vi "Test ThermotronDriver.vi"() -> (3 "gRPC Listening Port":i32)   [LabVIEW 2023]
uses:
  Plugin/ThermotronDriver/ThermotronDriver.lvclass
  <vilib>/ADAS Replay HIL/Template Node/Plugin/Template Node/Template Node.lvclass
  <vilib>/ADAS Replay HIL/ADAS Plugin Utilities/AdasLvTemplateSystemLog/AdasLvTemplateSystemLog.lvlib
  <vilib>/ADAS Replay HIL/Template Node/Plugin/Template Node/Common Configuration Params.ctl
  Plugin/ThermotronDriver/Configuration Params.ctl
panel:
  in  "Version":string="1.0"
  in  "Default Parameters":T1={"Common"={"Iteration Interval (s)"=0.001, "T0 (ns)"=0, "Priority"=100, "Processor"=-2, "Wait in Ready State"=TRUE}} {"Common"."Iteration Interval (s)" format="%#_13g"}
  out "# of errors":i32
  in  "stop":bool
  out "Errors":errorcluster[](array[cluster])
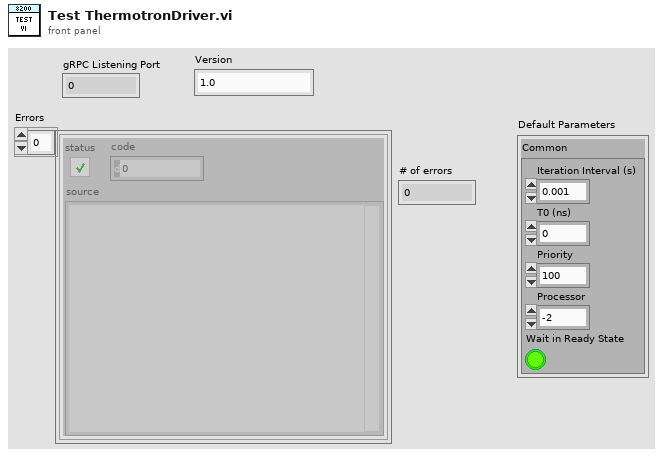
[diagram p1: front panel]
types:
  T1 = typedef "ThermotronDriver.lvlib/ThermotronDriver.lvclass/Configuration Params.ctl" = cluster{"Common":T2}
  T2 = typedef "Template Node.lvlib/Template Node.lvclass/Common Configuration Params.ctl" = cluster{"Iteration Interval (s)":dbl, "T0 (ns)":u64, "Priority":i32, "Processor":i32, "Wait in Ready State":bool}
  T3 = cluster{"Initial Setup":bool, "User Execute":bool, "Sequence Changed":bool, "Continuous Execution":bool, "Block Is Active":bool, "Animating Execution":bool}
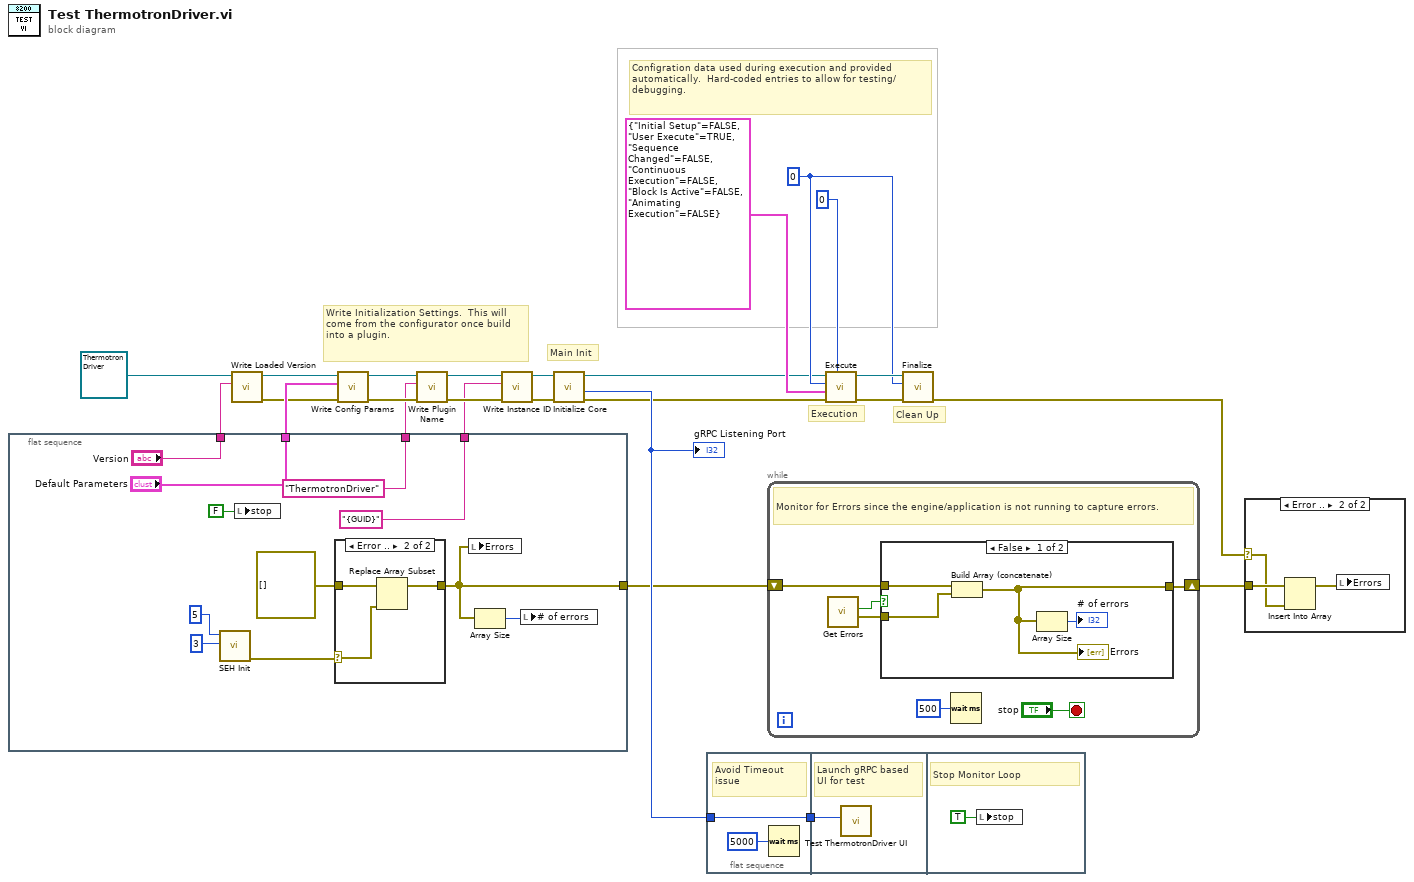
[diagram p0: block diagram]
diagram:
  w14 = u64 0 ("Handle")
  # "Clean Up"
  # "Execution"
  # "Configration data used during execution and provided automatically.  Hard-coded entries to allow for testing/debugging."
  # "Main Init"
  # "Write Initialization Settings.  This will come from the configurator once build into a plugin."
  n1 = flat-sequence {
    tunnel: ["ThermotronDriver" ("Plugin Name")] -> w17
    tunnel: ["{GUID}" ("Instance ID")] -> w16
    tunnel: ["Default Parameters"] -> w11
    tunnel: [w28] -> w8
    tunnel: ["Version"] -> w1
    frame #0 {
      n2 = call <userlib>:"SEH Init.vi"("Number of Priorities"=3, "Notifications per Priority"=5) -> ("error out"=w29:errorcluster)  [unwired: 9 in]
      n3 = local write "stop"(FALSE ("stop")) -> ()
      n4 = case shown="Error .." w29 {
        selector: w29 -> [_ w39]
        tunnel: errorcluster[] [] -> [w37 w40]
        tunnel: [w37 w38] -> w28
        frame No Error {
        }
        frame Error {
          n5 = Replace Array Subset(array=w40, new element=w39) -> (w38:errorcluster[])  [unwired: 1 in]
        }
      }
      n6 = local write "Errors"(w28) -> ()
      n7 = Array Size(array=w28) -> (size(s)=w27:i32)
      n8 = local write "# of errors"(w27) -> ()
    }
  }
  n9 = call <vilib>:"Write Loaded Version.vi"("Loaded Version"=w1, "Template Node in"=refnum<class "ThermotronDriver.lvclass"> refnum ("Test Node.lvlib:Test Node.lvclass")) -> ("error out"=w2:errorcluster, "Template Node out"=w3:refnum<class "ThermotronDriver.lvclass">)  [unwired: 8 in]
  n10 = call "Write Config Params.vi"("error in"=w2, "Default Parameters"=w11, "Node in"=w3) -> ("error out"=w23:errorcluster, "Node out"=w21:refnum<class "ThermotronDriver.lvclass">)  [unwired: 7 in]
  n11 = call <vilib>:"Write Plugin Name.vi"("error in"=w23, "Plugin Name"=w17, "Template Node in"=w21) -> ("error out"=w22:errorcluster, "Template Node out"=w19:refnum<class "ThermotronDriver.lvclass">)  [unwired: 7 in]
  n12 = call <vilib>:"Write Instance ID.vi"("error in"=w22, "Instance ID"=w16, "Template Node in"=w19) -> ("error out"=w20:errorcluster, "Template Node out"=w18:refnum<class "ThermotronDriver.lvclass">)  [unwired: 7 in]
  n13 = call <vilib>:"Initialize Core.vi"("error in"=w20, "Node in"=w18) -> ("error out"=w5:errorcluster, "gRPC Listening Port"=w10:i32, "Node out"=w9:refnum<class "ThermotronDriver.lvclass">)  [unwired: 7 in]
  "gRPC Listening Port" <- w10
  n14 = flat-sequence {
    tunnel: w10 -> [w42]
    tunnel: [w42] -> w4
    tunnel: w4 -> [w43]
    frame #0 {
      # "Avoid Timeout issue"
      n15 = Wait (ms)(milliseconds to wait=u32 5000) -> ()  [unwired: 1 out]
    }
    frame #1 {
      # "Launch gRPC based UI for test"
      n16 = call "Test ThermotronDriver UI.vi"("gRPC Port"=w43) -> ()  [unwired: 11 in]
    }
    frame #2 {
      # "Stop Monitor Loop"
      n17 = local write "stop"(TRUE ("stop")) -> ()
    }
  }
  n18 = while {
    shift-right: [w47] -> w7
    shift-left: w8 -> [w50]
    stop <- "stop" stop-if-true
    # "Monitor for Errors since the engine/application is not running to capture errors."
    n19 = call <vilib>:"Get Errors.vi"() -> ("Transmitted Errors"=w45:errorcluster[], "Empty?"=w46:bool)  [unwired: 9 in, 1 out]
    n20 = case shown="False" w46 {
      tunnel: w50 -> [w54 w55]
      tunnel: [w51 w55] -> w47
      tunnel: w45 -> [w53 _]
      frame False {
        n21 = Build Array (concatenate)(w54, w53) -> (w51:errorcluster[])
        "Errors" <- w51
        n22 = Array Size(array=w51) -> (size(s)=→"# of errors":i32)
      }
      frame True {
      }
    }
    n23 = Wait (ms)(milliseconds to wait=u32 500) -> ()  [unwired: 1 out]
  }
  n24 = call-dynamic "Execute.vi"("Pass Count"=u32 0, "error in (no error)"=w5, "Execute Reason"=T3 {"Initial Setup"=FALSE, "User Execute"=TRUE, "Sequence Changed"=FALSE, "Continuous Execution"=FALSE, "Block Is Active"=FALSE, "Animating Execution"=FALSE}, "Handle"=w14, "Node in"=w9) -> ("error out"=w13:errorcluster, "Node out"=w15:refnum<class "ThermotronDriver.lvclass">)  [unwired: 5 in]
  n25 = call-dynamic "Finalize.vi"("error in (no error)"=w13, "Handle"=w14, "Node in"=w15) -> ("error out"=w6:errorcluster)  [unwired: 7 in, 1 out]
  n26 = case shown="Error .." w6 {
    selector: w6 -> [_ w57]
    tunnel: w7 -> [_ w58]
    frame No Error {
    }
    frame Error {
      n27 = Insert Into Array(array=w58, new element=w57) -> (w56:errorcluster[])  [unwired: 1 in]
      n28 = local write "Errors"(w56) -> ()
    }
  }
